vi "DifferentialMotionMagicVelocityDutyCycle SetControl.vi"(0 "DeviceReference":T1, 1 "AverageVelocity":dbl, 2 "DifferentialPosition":dbl, 3 "EnableFOC":bool=TRUE, 4 "AverageSlot":i32, 5 "DifferentialSlot":i32=1, 6 "OverrideBrakeDurNeutral":bool, 7 "error in":errorcluster, 8 "LimitForwardMotion":bool, 9 "LimitReverseMotion":bool, 10 "IgnoreHardwareLimits":bool, 11 "IgnoreSoftwareLimits":bool, 12 "UseTimesync":bool, 18 "Update Frequency (Hz)":dbl=100.0) -> (20 "DeviceReference Out":T1, 27 "error out":errorcluster)   [LabVIEW 2025]
doc: "Requests Motion Magic® to target a final velocity using a motion profile, and PID to a differential position setpoint. This allows smooth transitions between velocity set points.\nMotion Magic® Velocity produces a motion profile in real-time while attempting to honor the specified Acceleration and (optional) Jerk. This control mode does not use the CruiseVelocity, Expo_kV, or Expo_kA configs.\nAcceleration and jerk are specified in the Motion Magic® persistent configuration values. If Jerk is set to zero, Motion Magic® will produce a trapezoidal acceleration profile.\nTarget velocity can also be changed on-the-fly and Motion Magic® will do its best to adjust the profile. This control mode is duty cycle based, so relevant closed-loop gains will use fractional duty cycle for the numerator: +1.0 represents full forward output."
uses:
  <vilib>/Rock Robotics/WPI/ThirdParty/Phoenix6/DeviceReference.ctl
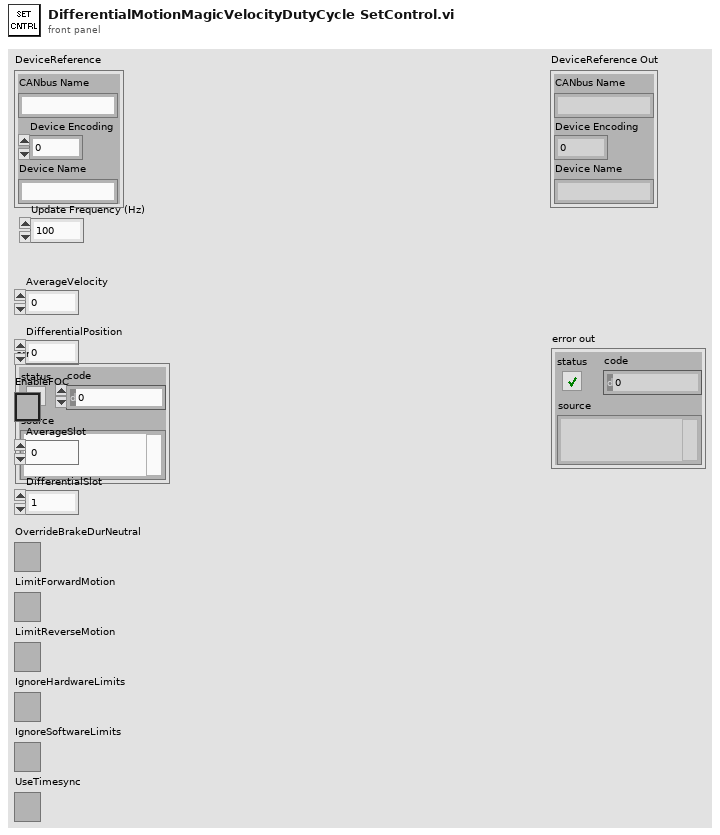
[diagram p1: front panel]
types:
  T1 = typedef "DeviceReference.ctl" = cluster{"CANbus Name":string, "Device Encoding":u32, "Device Name":string}
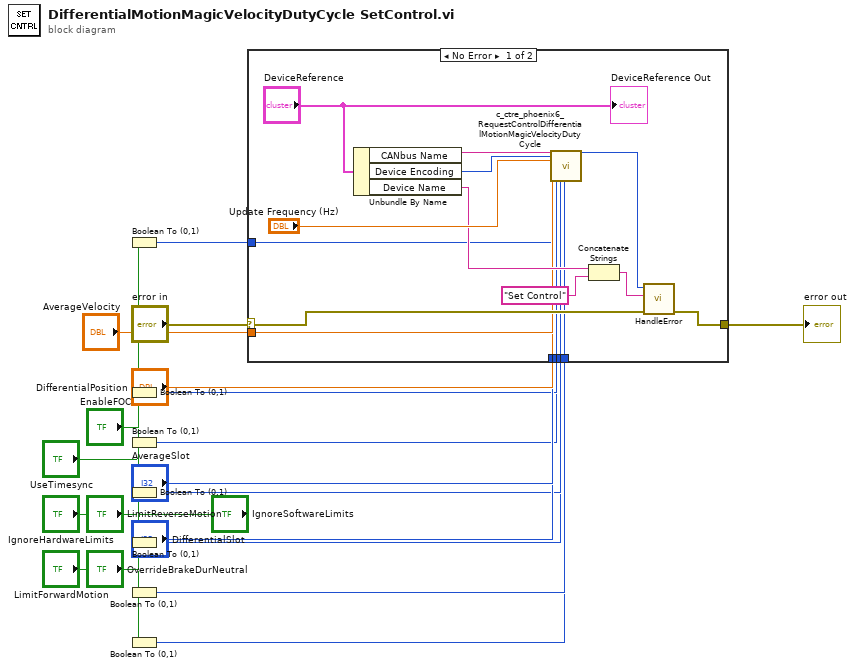
[diagram p0: block diagram]
diagram:
  n1 = Boolean To (0,1)(Boolean="EnableFOC") -> (0, 1=w15:i16)
  n2 = Boolean To (0,1)(Boolean="OverrideBrakeDurNeutral") -> (0, 1=w11:i16)
  n3 = Boolean To (0,1)(Boolean="LimitForwardMotion") -> (0, 1=w9:i16)
  n4 = Boolean To (0,1)(Boolean="LimitReverseMotion") -> (0, 1=w7:i16)
  n5 = Boolean To (0,1)(Boolean="IgnoreHardwareLimits") -> (0, 1=w5:i16)
  n6 = Boolean To (0,1)(Boolean="IgnoreSoftwareLimits") -> (0, 1=w3:i16)
  n7 = Boolean To (0,1)(Boolean="UseTimesync") -> (0, 1=w1:i16)
  n8 = case shown="No Error" "error in" {
    selector: "error in" -> [w36 w42]
    tunnel: [w35 w42] -> w19
    tunnel: "AverageVelocity" -> [w31 _]
    tunnel: "DifferentialPosition" -> [w30 _]
    tunnel: w15 -> [w29 _]
    tunnel: "AverageSlot" -> [w28 _]
    tunnel: "DifferentialSlot" -> [w27 _]
    tunnel: w11 -> [w26 _]
    tunnel: w9 -> [w25 _]
    tunnel: w7 -> [w24 _]
    tunnel: w5 -> [w23 _]
    tunnel: w3 -> [w22 _]
    tunnel: w1 -> [w21 _]
    frame No Error {
      n9 = Unbundle By Name("DeviceReference") -> ("CANbus Name"=w40:string, "Device Encoding"=w39:u32, "Device Name"=w34:string)
      n10 = call <vilib>:"c_ctre_phoenix6_RequestControlDifferentialMotionMagicVelocityDutyCycle.vi"("String 2"=w40, "Numeric 2"=w39, "Numeric 3"="Update Frequency (Hz)", "Numeric 4"=w31, "Numeric 5"=w30, "Numeric 6"=w29, "Numeric 7"=w28, "Numeric 8"=w27, "Numeric 9"=w26, "Numeric 10"=w25, "Numeric 11"=w24, "Numeric 12"=w23, "Numeric 13"=w22, "Numeric 14"=w21) -> ("Numeric"=w37:i32)  [unwired: 12 in, 1 out]
      n11 = Concatenate Strings(w34, "Set Control" ("origin")) -> (w32:string)
      n12 = call <vilib>:"HandleError.vi"("error in"=w36, "origin"=w32, "Status"=w37) -> ("error out"=w35:errorcluster)  [unwired: 8 in]
      "DeviceReference Out" <- "DeviceReference"
    }
    frame Error {
    }
  }
  "error out" <- w19
